vi "libssh2_exit.vi"(8 "error in (no error)":errorcluster) -> (0 "error out":errorcluster)   [LabVIEW 2013, in "libssh2.lvlib"]
doc: "Exits libssh2 and frees all memory used internally."
uses:
  libssh2.lvlib
  Global Settings.vi
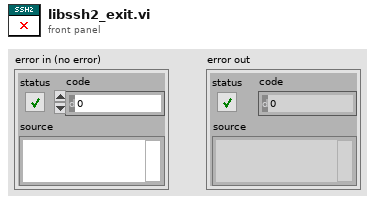
[diagram p1: front panel]
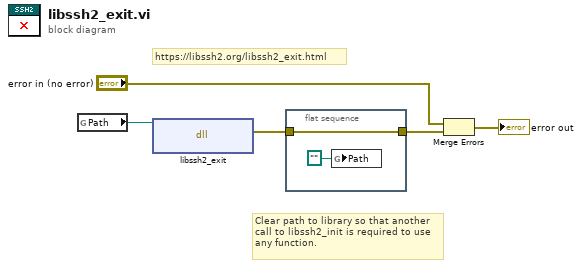
[diagram p0: block diagram]
diagram:
  # "Clear path to library so that another\ncall to libssh2_init is required to use\nany function."
  # "https://libssh2.org/libssh2_exit.html"
  n1 = global read "Global Settings.vi" "Path"() -> (w3:path)
  n2 = dll-call lib="C:/Users/pasca/source/repos/libssh2-labview/libssh2/libssh2**.*" fn="libssh2_exit"(path in=w3) -> (error out=w1:errorcluster)  [unwired: 3 in, 1 out]
  n3 = flat-sequence {
    tunnel: [w7] -> w2
    tunnel: w1 -> [w7]
    frame #0 {
      n4 = global write "Global Settings.vi" "Path"(path "") -> ()
    }
  }
  n5 = Merge Errors("error in (no error)", w2) -> (→"error out":errorcluster)
